vi "Hardware In - NI 9755-1 (NOx).vi"(11 "FPGA Ref":T1) -> ()   [LabVIEW 2015, in "ECS-RT.lvlib"]
uses:
  ECS-RT.lvlib
  Typedefs/FPGA Refs/Generic FPGA Ref.ctl
  <vilib>/Utility/error.llb/Error Cluster From Error Code.vi
  <vilib>/rvi/errors/niLvFpgaAdjustHostInterfaceError.vi
  <vilib>/rvi/interface/nirviReadWriteControl/nirviReadWriteControl.xnode
  <vilib>/rvi/interface/Simulation/niFpgaSimulationCallBeginRW.vi
  NiFpgaLv.dll
  ECS-Shared.lvlib
panel:
  out "NOx1 Data":T2={"NOx (ppm)"=0, "O2 (%)"=0.0, "Sensor Supply Status"=3, "Sensor Temperature Status"=12, "NOx Signal Status"=48, "O2 Signal Status"=192, "Heater Mode Status"=96, "Heater Circuit Status"=31, "NOx Circuit Status"=31, "O2 Circuit Status"=31, "NOx Sensor Module Present"=FALSE} {"Heater Mode Status" items=["AUTO MODE"=0, "HEATUP SLOPE 3 OR 4"=32, "HEATUP SLOPE 1 OR 2"=64, "HEATER OFF / PREHEAT"=96]; "O2 Circuit Status" items=["OPEN WIRE"=3, "SHORT CIRCUIT"=5, "NO ERROR"=31]; "NOx Circuit Status" items=["OPEN WIRE"=3, "SHORT CIRCUIT"=5, "NO ERROR"=31]; "Heater Circuit Status" items=["OPEN WIRE"=3, "SHORT CIRCUIT"=5, "NO ERROR"=31]; "Sensor Temperature Status" items=["NOT AT TEMPERATURE"=0, "AT TEMPERATURE"=4, "ERROR"=8, "NOT AVAILABLE"=12]; "O2 Signal Status" items=["NOT VALID"=0, "VALID"=64, "ERROR"=128, "NOT AVAILABLE"=192]; "NOx Signal Status" items=["NOT VALID"=0, "VALID"=16, "ERROR"=32, "NOT AVAILABLE"=48]; "Sensor Supply Status" items=["NOT IN RANGE", "SUPPLY IN RANGE", "ERROR", "NOT AVAILABLE"]}
  out "NOx2 Data":T2={"NOx (ppm)"=0, "O2 (%)"=0.0, "Sensor Supply Status"=3, "Sensor Temperature Status"=12, "NOx Signal Status"=48, "O2 Signal Status"=192, "Heater Mode Status"=96, "Heater Circuit Status"=31, "NOx Circuit Status"=31, "O2 Circuit Status"=31, "NOx Sensor Module Present"=FALSE} {"Heater Mode Status" items=["AUTO MODE"=0, "HEATUP SLOPE 3 OR 4"=32, "HEATUP SLOPE 1 OR 2"=64, "HEATER OFF / PREHEAT"=96]; "O2 Circuit Status" items=["OPEN WIRE"=3, "SHORT CIRCUIT"=5, "NO ERROR"=31]; "NOx Circuit Status" items=["OPEN WIRE"=3, "SHORT CIRCUIT"=5, "NO ERROR"=31]; "Heater Circuit Status" items=["OPEN WIRE"=3, "SHORT CIRCUIT"=5, "NO ERROR"=31]; "Sensor Temperature Status" items=["NOT AT TEMPERATURE"=0, "AT TEMPERATURE"=4, "ERROR"=8, "NOT AVAILABLE"=12]; "O2 Signal Status" items=["NOT VALID"=0, "VALID"=64, "ERROR"=128, "NOT AVAILABLE"=192]; "NOx Signal Status" items=["NOT VALID"=0, "VALID"=16, "ERROR"=32, "NOT AVAILABLE"=48]; "Sensor Supply Status" items=["NOT IN RANGE", "SUPPLY IN RANGE", "ERROR", "NOT AVAILABLE"]}
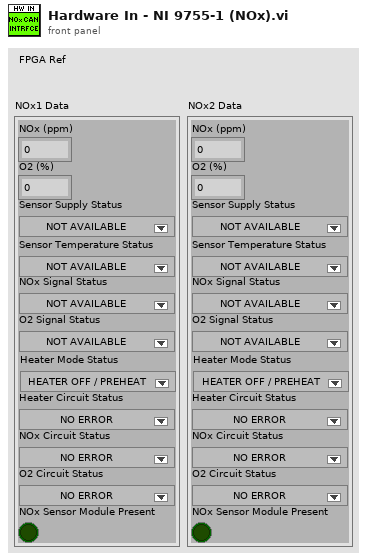
[diagram p1: front panel]
types:
  T1 = typedef "ECS-Shared.lvlib/Generic FPGA Ref.ctl" = refnum<k20>
  T2 = cluster{"NOx (ppm)":i16, "O2 (%)":sgl, "Sensor Supply Status":u8, "Sensor Temperature Status":u8, "NOx Signal Status":u8, "O2 Signal Status":u8, "Heater Mode Status":u8, "Heater Circuit Status":u8, "NOx Circuit Status":u8, "O2 Circuit Status":u8, "NOx Sensor Module Present":bool}
  T3 = cluster{"NOx (bits)":u16, "O2 (bits)":u16, "Sensor Supply Status":u8, "Sensor Temperature Status":u8, "NOx Signal Status":u8, "O2 Signal Status":u8, "Heater Mode Status":u8, "Heater Circuit Status":u8, "NOx Circuit Status":u8, "O2 Circuit Status":u8, "NOx Sensor Module Present":bool}
  T4 = cluster{"NOx (ppm)":sgl, "O2 (%)":sgl, "Sensor Supply Status":u8, "Sensor Temperature Status":u8, "NOx Signal Status":u8, "O2 Signal Status":u8, "Heater Mode Status":u8, "Heater Circuit Status":u8, "NOx Circuit Status":u8, "O2 Circuit Status":u8, "NOx Sensor Module Present":bool}
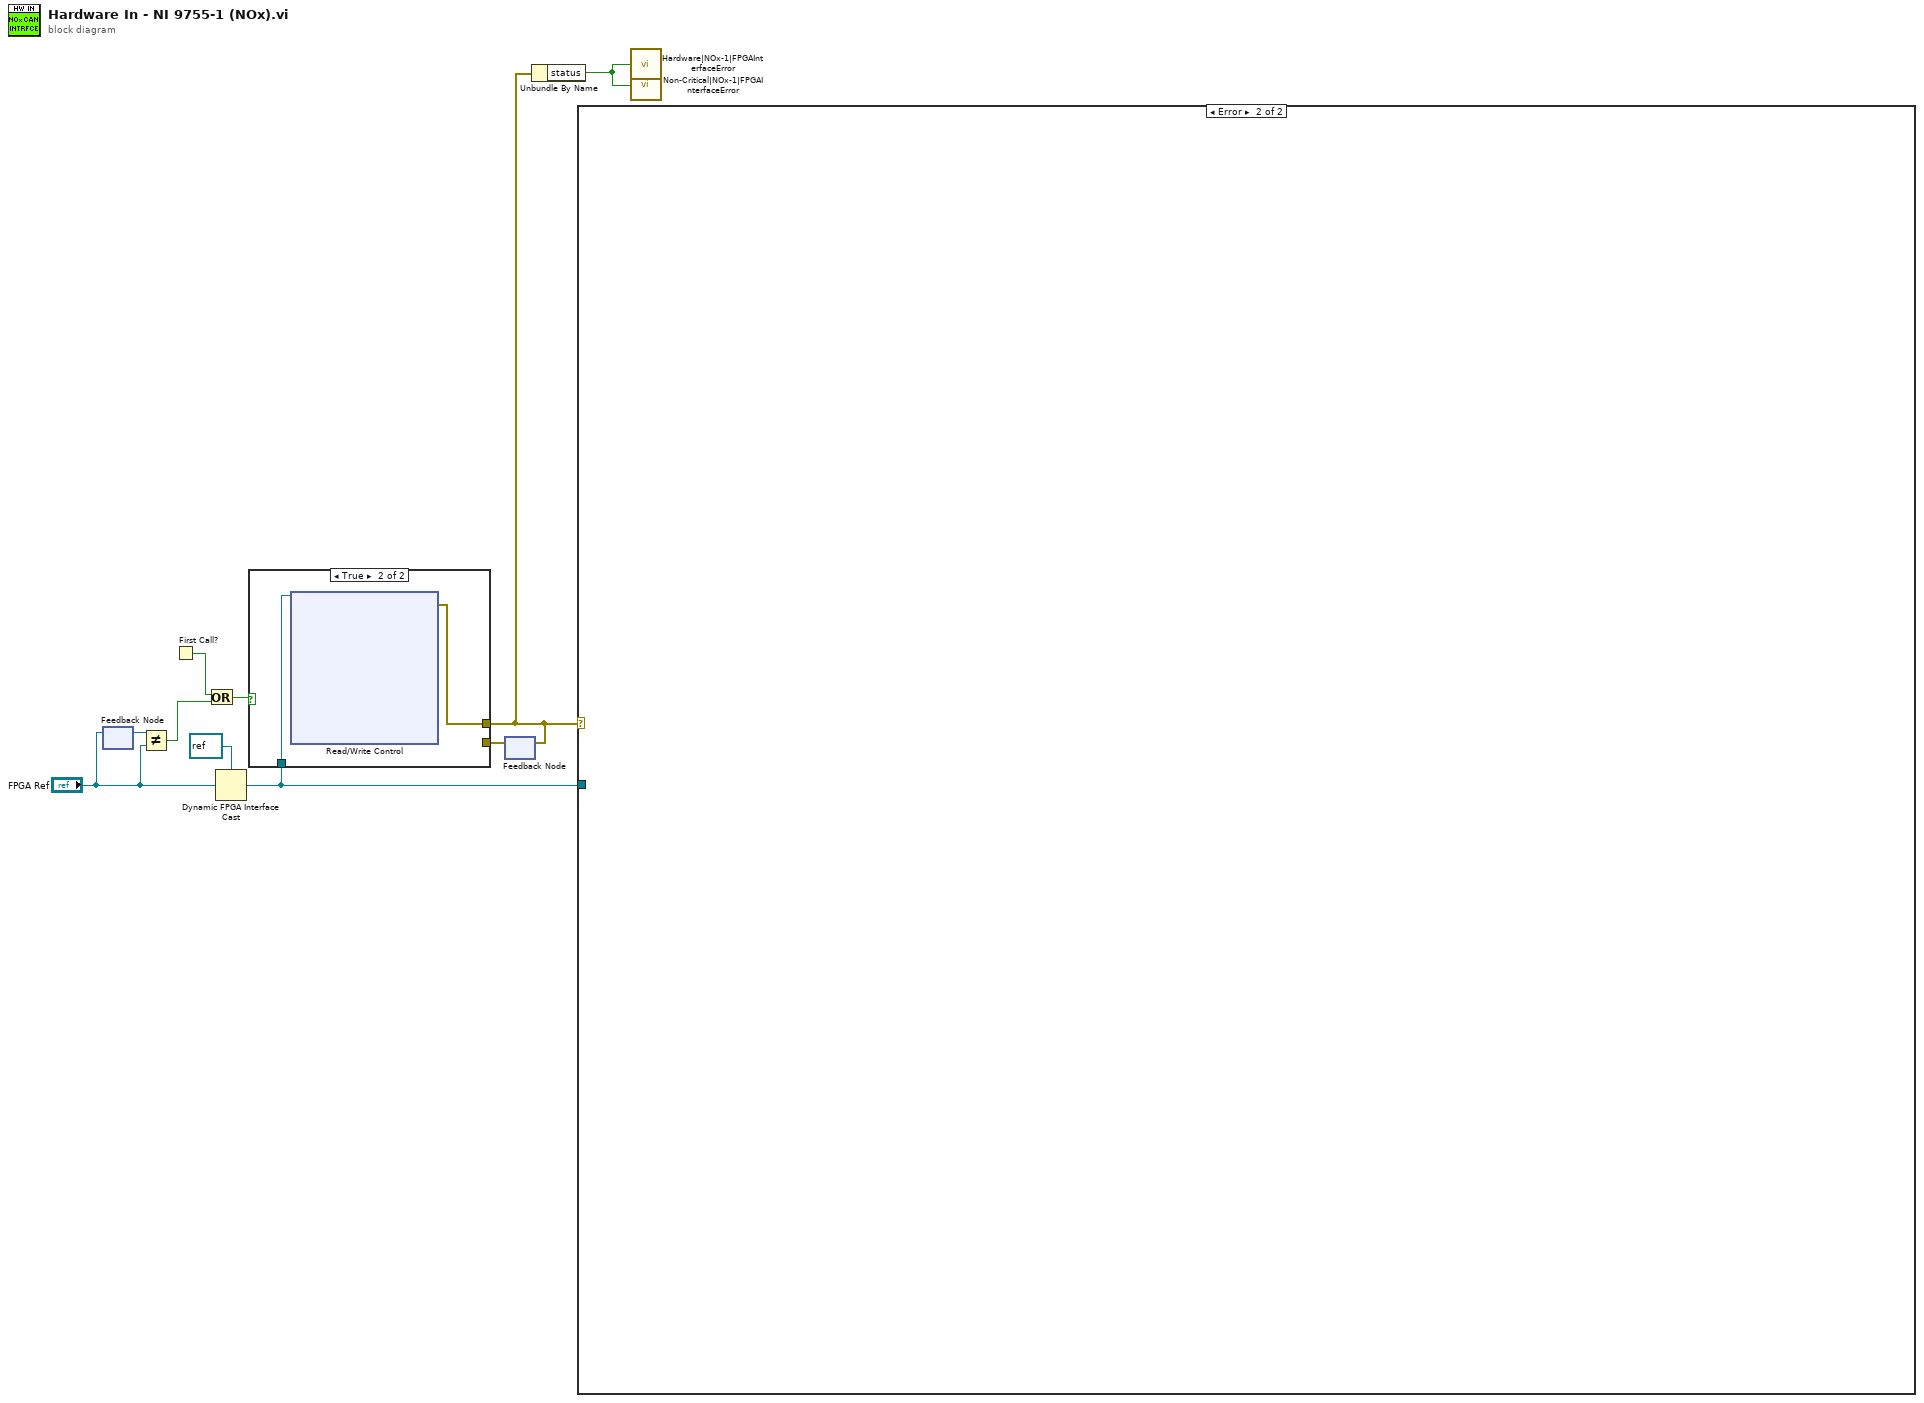
[diagram p0: block diagram]
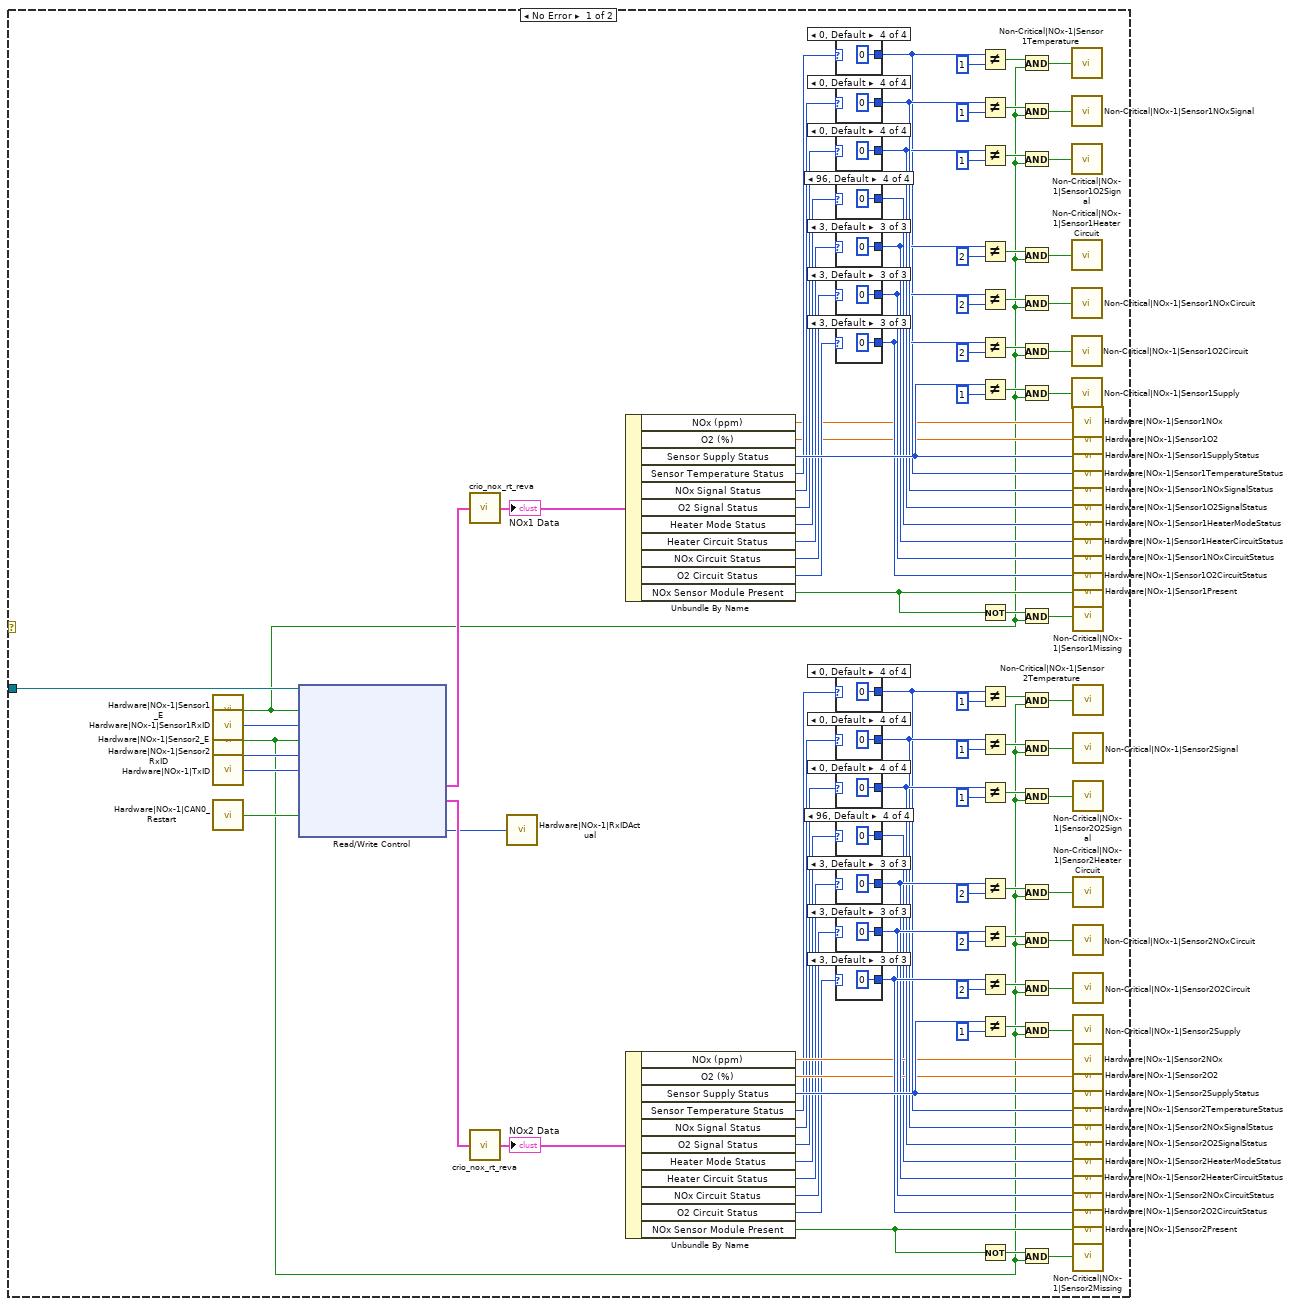
[diagram p3: hidden frame]
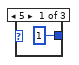
[diagram p4: hidden frame]
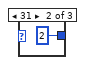
[diagram p5: hidden frame]
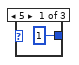
[diagram p6: hidden frame]
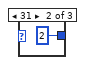
[diagram p7: hidden frame]
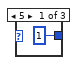
[diagram p8: hidden frame]
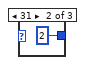
[diagram p9: hidden frame]
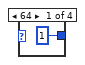
[diagram p10: hidden frame]
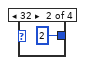
[diagram p11: hidden frame]
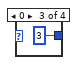
[diagram p12: hidden frame]
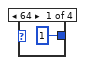
[diagram p13: hidden frame]
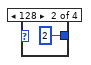
[diagram p14: hidden frame]
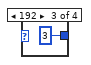
[diagram p15: hidden frame]
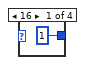
[diagram p16: hidden frame]
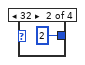
[diagram p17: hidden frame]
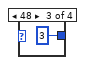
[diagram p18: hidden frame]
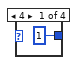
[diagram p19: hidden frame]
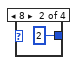
[diagram p20: hidden frame]
diagram:
  n1 = feedback #1() -> (w9:T1)  [unwired: 1 in]
  n2 = feedback-in #1("FPGA Ref") -> ()
  n3 = Not Equal?(x=w9, y="FPGA Ref") -> (x != y?=w10:bool)
  n4 = First Call?() -> (First Call?: T/F=w8:bool)
  n5 = Or(x=w8, y=w10) -> (x .or. y?=w7:bool)
  n6 = Dynamic FPGA Interface Cast(Session In=refnum<k20> refnum ("FPGA VI Reference Out"), Type="FPGA Ref") -> (Session Out=w3:refnum<k20>)
  n7 = feedback #2() -> (w6:errorcluster)  [unwired: 1 in]
  n8 = case shown="True" w7 {
    tunnel: [w11 w13] -> w2
    tunnel: w6 -> [w11 _]
    tunnel: w3 -> [_ w12]
    frame False {
    }
    frame True {
      n9 = xnode "Read/Write Control"("FPGA VI Reference In"=w12) -> ("error out"=w13:errorcluster)  [unwired: 7 in, 4 out]
    }
  }
  n10 = feedback-in #2(w2) -> ()
  n11 = Unbundle By Name(w2) -> ("status"=w1:bool)
  n12 = case shown="Error" w2 {
    tunnel: w3 -> [w49 _]
    frame No Error {
      n13 = call "Hardware|NOx-1|Sensor1_E"() -> ("Value"=w15:bool)
      n14 = call "Hardware|NOx-1|Sensor1RxID"() -> ("Value"=w107:u32)
      n15 = call "Hardware|NOx-1|Sensor2_E"() -> ("Value"=w32:bool)
      n16 = call "Hardware|NOx-1|Sensor2RxID"() -> ("Value"=w106:u32)
      n17 = call "Hardware|NOx-1|TxID"() -> ("Value"=w105:u32)
      n18 = call "Hardware|NOx-1|CAN0_Restart"() -> ("Value"=w104:bool)
      n19 = xnode "Read/Write Control"("FPGA VI Reference In"=w49, "9755-1.Sensor 1 Enable"=w15, "9755-1.RxID 1"=w107, "9755-1.Sensor 2 Enable"=w32, "9755-1.RxID 2"=w106, "9755-1.TxID"=w105, "9755-1.CAN0 Restart"=w104) -> ("9755-1.NOxSensorData 1"=w50:T3, "9755-1.NOxSensorData 2"=w51:T3, "9755-1.RxID Actual"=w14:u32)  [unwired: 1 in, 2 out]
      n20 = call <vilib>:"crio_nox_rt_reva.vi"("NOxSensorDataFromFPGA"=w50) -> ("NOxSensorData"=w61:T4)
      "NOx1 Data" <- w61
      n21 = call <vilib>:"crio_nox_rt_reva.vi"("NOxSensorDataFromFPGA"=w51) -> ("NOxSensorData"=w62:T4)
      "NOx2 Data" <- w62
      n22 = call "Hardware|NOx-1|RxIDActual"("Value"=w14) -> ()
      n23 = Unbundle By Name(w61) -> ("NOx (ppm)"=w52:sgl, "O2 (%)"=w53:sgl, "Sensor Supply Status"=w87:u8, "Sensor Temperature Status"=w54:u8, "NOx Signal Status"=w55:u8, "O2 Signal Status"=w56:u8, "Heater Mode Status"=w57:u8, "Heater Circuit Status"=w58:u8, "NOx Circuit Status"=w59:u8, "O2 Circuit Status"=w60:u8, "NOx Sensor Module Present"=w88:bool)
      n24 = Unbundle By Name(w62) -> ("NOx (ppm)"=w72:sgl, "O2 (%)"=w71:sgl, "Sensor Supply Status"=w102:u8, "Sensor Temperature Status"=w70:u8, "NOx Signal Status"=w69:u8, "O2 Signal Status"=w68:u8, "Heater Mode Status"=w66:u8, "Heater Circuit Status"=w65:u8, "NOx Circuit Status"=w64:u8, "O2 Circuit Status"=w63:u8, "NOx Sensor Module Present"=w103:bool)
      n25 = case shown="0, Default" w54 {
        tunnel: [1 2 3 0] -> w73
        frame 4 {
        }
        frame 8 {
        }
        frame 12 {
        }
        frame 0, Default {
        }
      }
      n26 = case shown="0, Default" w55 {
        tunnel: [1 2 3 0] -> w85
        frame 16 {
        }
        frame 32 {
        }
        frame 48 {
        }
        frame 0, Default {
        }
      }
      n27 = case shown="0, Default" w56 {
        tunnel: [1 2 3 0] -> w84
        frame 64 {
        }
        frame 128 {
        }
        frame 192 {
        }
        frame 0, Default {
        }
      }
      n28 = case shown="96, Default" w57 {
        tunnel: [1 2 3 0] -> w83
        frame 64 {
        }
        frame 32 {
        }
        frame 0 {
        }
        frame 96, Default {
        }
      }
      n29 = case shown="3, Default" w58 {
        tunnel: [1 2 0] -> w82
        frame 5 {
        }
        frame 31 {
        }
        frame 3, Default {
        }
      }
      n30 = case shown="3, Default" w59 {
        tunnel: [1 2 0] -> w81
        frame 5 {
        }
        frame 31 {
        }
        frame 3, Default {
        }
      }
      n31 = case shown="3, Default" w60 {
        tunnel: [1 2 0] -> w80
        frame 5 {
        }
        frame 31 {
        }
        frame 3, Default {
        }
      }
      n32 = case shown="0, Default" w70 {
        tunnel: [1 2 3 0] -> w96
        frame 4 {
        }
        frame 8 {
        }
        frame 12 {
        }
        frame 0, Default {
        }
      }
      n33 = case shown="0, Default" w69 {
        tunnel: [1 2 3 0] -> w97
        frame 16 {
        }
        frame 32 {
        }
        frame 48 {
        }
        frame 0, Default {
        }
      }
      n34 = case shown="0, Default" w68 {
        tunnel: [1 2 3 0] -> w98
        frame 64 {
        }
        frame 128 {
        }
        frame 192 {
        }
        frame 0, Default {
        }
      }
      n35 = case shown="96, Default" w66 {
        tunnel: [1 2 3 0] -> w67
        frame 64 {
        }
        frame 32 {
        }
        frame 0 {
        }
        frame 96, Default {
        }
      }
      n36 = case shown="3, Default" w65 {
        tunnel: [1 2 0] -> w99
        frame 5 {
        }
        frame 31 {
        }
        frame 3, Default {
        }
      }
      n37 = case shown="3, Default" w64 {
        tunnel: [1 2 0] -> w100
        frame 5 {
        }
        frame 31 {
        }
        frame 3, Default {
        }
      }
      n38 = case shown="3, Default" w63 {
        tunnel: [1 2 0] -> w101
        frame 5 {
        }
        frame 31 {
        }
        frame 3, Default {
        }
      }
      n39 = Not Equal?(x=w73, y=1) -> (x != y?=w30:bool)
      n40 = Not Equal?(x=w85, y=1) -> (x != y?=w21:bool)
      n41 = Not Equal?(x=w84, y=1) -> (x != y?=w20:bool)
      n42 = Not Equal?(x=w82, y=2) -> (x != y?=w19:bool)
      n43 = Not Equal?(x=w81, y=2) -> (x != y?=w18:bool)
      n44 = Not Equal?(x=w80, y=2) -> (x != y?=w17:bool)
      n45 = Not Equal?(x=w87, y=1) -> (x != y?=w16:bool)
      n46 = Not(x=w88) -> (.not. x?=w28:bool)
      n47 = Not Equal?(x=w96, y=1) -> (x != y?=w40:bool)
      n48 = Not Equal?(x=w97, y=1) -> (x != y?=w39:bool)
      n49 = Not Equal?(x=w98, y=1) -> (x != y?=w38:bool)
      n50 = Not Equal?(x=w99, y=2) -> (x != y?=w37:bool)
      n51 = Not Equal?(x=w100, y=2) -> (x != y?=w36:bool)
      n52 = Not Equal?(x=w101, y=2) -> (x != y?=w35:bool)
      n53 = Not Equal?(x=w102, y=1) -> (x != y?=w34:bool)
      n54 = Not(x=w103) -> (.not. x?=w33:bool)
      n55 = And(x=w30, y=w15) -> (x .and. y?=w31:bool)
      n56 = And(x=w21, y=w15) -> (x .and. y?=w22:bool)
      n57 = And(x=w20, y=w15) -> (x .and. y?=w23:bool)
      n58 = And(x=w19, y=w15) -> (x .and. y?=w24:bool)
      n59 = And(x=w18, y=w15) -> (x .and. y?=w25:bool)
      n60 = And(x=w17, y=w15) -> (x .and. y?=w27:bool)
      n61 = And(x=w16, y=w15) -> (x .and. y?=w26:bool)
      n62 = And(x=w28, y=w15) -> (x .and. y?=w29:bool)
      n63 = And(x=w40, y=w32) -> (x .and. y?=w48:bool)
      n64 = And(x=w39, y=w32) -> (x .and. y?=w47:bool)
      n65 = And(x=w38, y=w32) -> (x .and. y?=w46:bool)
      n66 = And(x=w37, y=w32) -> (x .and. y?=w45:bool)
      n67 = And(x=w36, y=w32) -> (x .and. y?=w44:bool)
      n68 = And(x=w35, y=w32) -> (x .and. y?=w43:bool)
      n69 = And(x=w34, y=w32) -> (x .and. y?=w42:bool)
      n70 = And(x=w33, y=w32) -> (x .and. y?=w41:bool)
      n71 = call "Non-Critical|NOx-1|Sensor1Temperature"("Fault"=w31) -> ()  [unwired: 2 in]
      n72 = call "Non-Critical|NOx-1|Sensor1NOxSignal"("Fault"=w22) -> ()  [unwired: 2 in]
      n73 = call "Non-Critical|NOx-1|Sensor1O2Signal"("Fault"=w23) -> ()  [unwired: 2 in]
      n74 = call "Non-Critical|NOx-1|Sensor1HeaterCircuit"("Fault"=w24) -> ()  [unwired: 2 in]
      n75 = call "Non-Critical|NOx-1|Sensor1NOxCircuit"("Fault"=w25) -> ()  [unwired: 2 in]
      n76 = call "Non-Critical|NOx-1|Sensor1O2Circuit"("Fault"=w27) -> ()  [unwired: 2 in]
      n77 = call "Non-Critical|NOx-1|Sensor1Supply"("Fault"=w26) -> ()  [unwired: 2 in]
      n78 = call "Hardware|NOx-1|Sensor1NOx"("Value"=w52) -> ()
      n79 = call "Hardware|NOx-1|Sensor1O2"("Value"=w53) -> ()
      n80 = call "Hardware|NOx-1|Sensor1SupplyStatus"("Value"=w87) -> ()
      n81 = call "Hardware|NOx-1|Sensor1TemperatureStatus"("Value"=w73) -> ()
      n82 = call "Hardware|NOx-1|Sensor1NOxSignalStatus"("Value"=w85) -> ()
      n83 = call "Hardware|NOx-1|Sensor1O2SignalStatus"("Value"=w84) -> ()
      n84 = call "Hardware|NOx-1|Sensor1HeaterModeStatus"("Value"=w83) -> ()
      n85 = call "Hardware|NOx-1|Sensor1HeaterCircuitStatus"("Value"=w82) -> ()
      n86 = call "Hardware|NOx-1|Sensor1NOxCircuitStatus"("Value"=w81) -> ()
      n87 = call "Hardware|NOx-1|Sensor1O2CircuitStatus"("Value"=w80) -> ()
      n88 = call "Hardware|NOx-1|Sensor1Present"("Value"=w88) -> ()
      n89 = call "Non-Critical|NOx-1|Sensor1Missing"("Fault"=w29) -> ()  [unwired: 2 in]
      n90 = call "Non-Critical|NOx-1|Sensor2Temperature"("Fault"=w48) -> ()  [unwired: 2 in]
      n91 = call "Non-Critical|NOx-1|Sensor2Signal"("Fault"=w47) -> ()  [unwired: 2 in]
      n92 = call "Non-Critical|NOx-1|Sensor2O2Signal"("Fault"=w46) -> ()  [unwired: 2 in]
      n93 = call "Non-Critical|NOx-1|Sensor2HeaterCircuit"("Fault"=w45) -> ()  [unwired: 2 in]
      n94 = call "Non-Critical|NOx-1|Sensor2NOxCircuit"("Fault"=w44) -> ()  [unwired: 2 in]
      n95 = call "Non-Critical|NOx-1|Sensor2O2Circuit"("Fault"=w43) -> ()  [unwired: 2 in]
      n96 = call "Non-Critical|NOx-1|Sensor2Supply"("Fault"=w42) -> ()  [unwired: 2 in]
      n97 = call "Hardware|NOx-1|Sensor2NOx"("Value"=w72) -> ()
      n98 = call "Hardware|NOx-1|Sensor2O2"("Value"=w71) -> ()
      n99 = call "Hardware|NOx-1|Sensor2SupplyStatus"("Value"=w102) -> ()
      n100 = call "Hardware|NOx-1|Sensor2TemperatureStatus"("Value"=w96) -> ()
      n101 = call "Hardware|NOx-1|Sensor2NOxSignalStatus"("Value"=w97) -> ()
      n102 = call "Hardware|NOx-1|Sensor2O2SignalStatus"("Value"=w98) -> ()
      n103 = call "Hardware|NOx-1|Sensor2HeaterModeStatus"("Value"=w67) -> ()
      n104 = call "Hardware|NOx-1|Sensor2HeaterCircuitStatus"("Value"=w99) -> ()
      n105 = call "Hardware|NOx-1|Sensor2NOxCircuitStatus"("Value"=w100) -> ()
      n106 = call "Hardware|NOx-1|Sensor2O2CircuitStatus"("Value"=w101) -> ()
      n107 = call "Hardware|NOx-1|Sensor2Present"("Value"=w103) -> ()
      n108 = call "Non-Critical|NOx-1|Sensor2Missing"("Fault"=w41) -> ()  [unwired: 2 in]
    }
    frame Error {
    }
  }
  n109 = call "Hardware|NOx-1|FPGAInterfaceError"("Value"=w1) -> ()
  n110 = call "Non-Critical|NOx-1|FPGAInterfaceError"("Fault"=w1) -> ()  [unwired: 2 in]
